vi "Decompose Lib-Class-Name.vi"(11 "Qualified Name":string) -> (0 "VI/Control":string, 1 "className":string, 2 "libName":string, 3 "libName w/ext":string, 5 "ppl":bool)   [LabVIEW 2021, in "smo.lvlib" / "SMO.lvclass"]
uses:
  SMO.lvclass
  <vilib>/regexp/Match Regular Expression.xnode
  SMO.lvclass/SMO.ctl
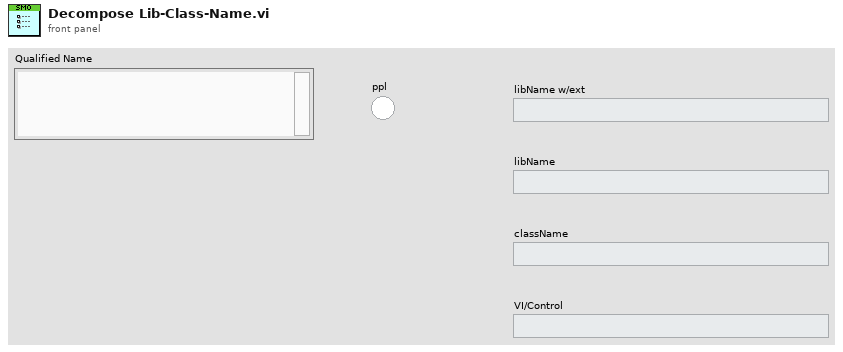
[diagram p1: front panel]
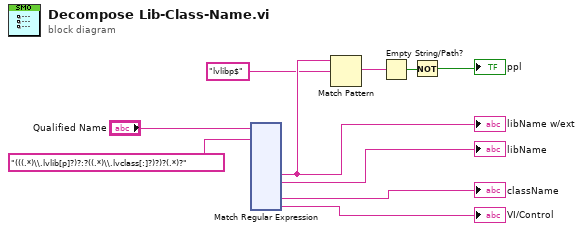
[diagram p0: block diagram]
diagram:
  n1 = xnode "Match Regular Expression"("input string"="Qualified Name", "regular expression"="(((.*)\\.lvlib[p]?)?:?((.*)\\.lvclass[:]?)?)?(.*)?") -> ("submatch 2"=w7:string, "submatch 3"=→"libName":string, "submatch 5"=→"className":string, "submatch 6"=→"VI/Control":string)  [unwired: 4 in, 7 out]
  "libName w/ext" <- w7
  n2 = Match Pattern(string=w7, regular expression="lvlibp$") -> (match substring=w5:string)  [unwired: 1 in, 3 out]
  n3 = Empty String/Path?(string/path=w5) -> (empty?=w4:bool)
  n4 = Not(x=w4) -> (.not. x?=→"ppl":bool)
